vi "Activate Motor.vi"(0 "reference in":refnum<class "PM_Group.lvclass">, 5 "Active Motor":T1, 11 "error in (no error)":errorcluster) -> (4 "reference out":refnum<class "PM_Group.lvclass">, 15 "error out":errorcluster)   [LabVIEW 2019, in "PM_Group.lvclass"]
uses:
  PM_Group.lvclass
  D:/GIT H4000/H4000/src/Device_class/Device.lvclass
  TypeDef/Active Motor.ctl
  TypeDef/Motor N.ctl
  PM_Group.lvclass/PM_Group.ctl
  FPGA/TypeDef/DO index.ctl
  Device_class/Device.lvclass/Device.ctl
  FPGA_API_class/FPGA API.lvclass
  Engine_1DO_2DI_class/Engine_1DO_2DI.lvclass
  Device_class/Device.lvclass
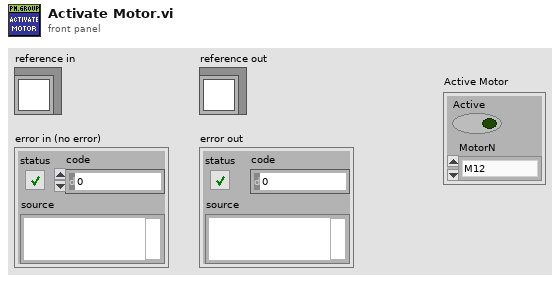
[diagram p1: front panel]
types:
  T1 = typedef "Active Motor.ctl" = cluster{"Active":bool, "MotorN":T2}
  T2 = typedef "Motor N.ctl" = enum16{"M12", "M21", "M24"}
  T3 = typedef "DO index.ctl" = u8
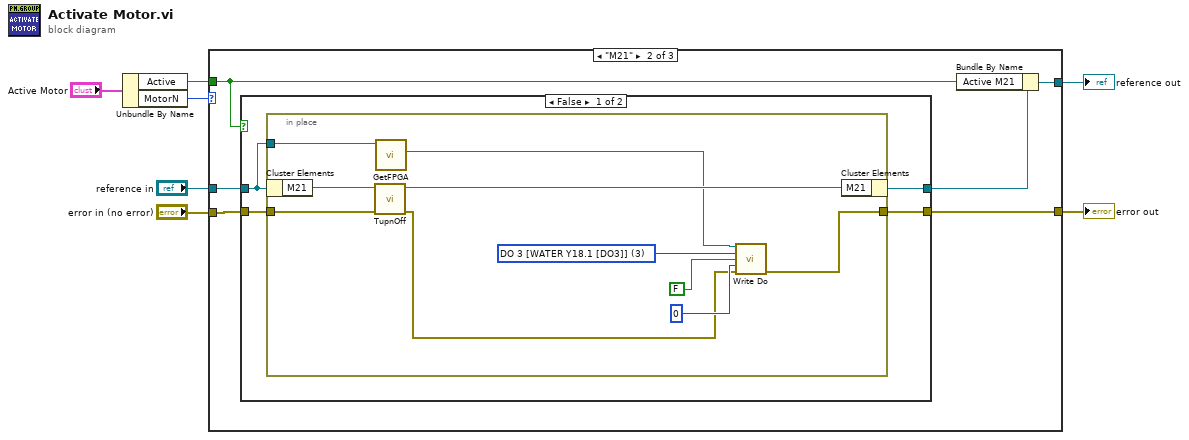
[diagram p0: block diagram]
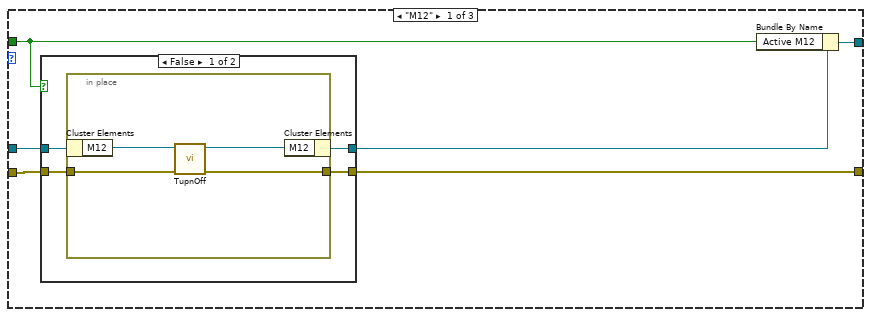
[diagram p2: hidden frame]
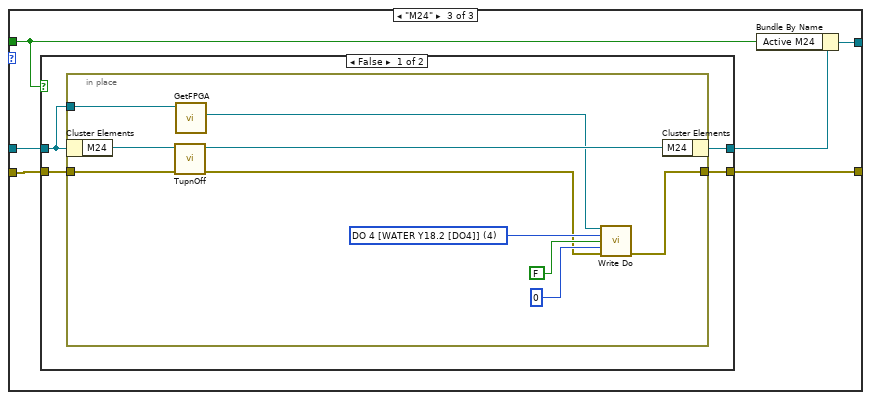
[diagram p5: hidden frame]
diagram:
  n1 = Unbundle By Name("Active Motor") -> ("Active"=w2:bool, "MotorN"=w1:T2)
  n2 = case shown="\"M21\"" w1 {
    tunnel: [w13 w29 w51] -> w7
    tunnel: "error in (no error)" -> [w12 w28 w50]
    tunnel: "reference in" -> [w10 w26 w48]
    tunnel: [w9 w25 w47] -> w4
    tunnel: w2 -> [w8 w24 w46]
    frame "M12" {
      n3 = case shown="False" w8 {
        tunnel: [w17 w22] -> w13
        tunnel: w12 -> [w16 w22]
        tunnel: [w15 w23] -> w11
        tunnel: w10 -> [w14 w23]
        frame False {
          n4 = in-place {
            in-place-border: w16 -> [w19]
            in-place-border: [w18] -> w17
            n5 = in-place-cluster #1(w14) -> ("M12"=w21:refnum<class "Engine_1DO_2DI.lvclass">)
            n6 = call "TupnOff.vi"("error in (no error)"=w19, "Pump_1AI_1DO_2DI in"=w21) -> ("error out"=w18:errorcluster, "Pump_1AI_1DO_2DI out"=w20:refnum<class "Engine_1DO_2DI.lvclass">)  [unwired: 8 in]
            n7 = in-place-cluster #1("M12"=w20) -> (w15:refnum<class "PM_Group.lvclass">)
          }
        }
        frame True {
        }
      }
      n8 = Bundle By Name(cluster=w11, "Active M12"=w8) -> (w9:refnum<class "PM_Group.lvclass">)
    }
    frame "M21" {
      n9 = case shown="False" w24 {
        tunnel: [w33 w44] -> w29
        tunnel: w28 -> [w32 w44]
        tunnel: [w31 w45] -> w27
        tunnel: w26 -> [w30 w45]
        frame False {
          n10 = in-place {
            in-place-border: w32 -> [w41]
            in-place-border: [w36] -> w33
            in-place-border: w30 -> [w35]
            w40 = T3 3 items=["DO 0 [KP1 [DO 0]]", "DO 1 [ON KP2 [DO 1]]", "DO 2 [ON KP3 [DO 2]]", "DO 3 [WATER Y18.1 [DO3]]", "DO 4 [WATER Y18.2 [DO4]]", "DO 5 [KP6 Y29.1 33.7]", "DO 6 [KP7 Y29.2 33.8]", "DO 7 [KP8 Y29.3 33.9]", "DO 8 [KP9 Y29.4  33.12]", "DO 9 [KP10 Y29.5 33.1]", "DO 10 [KP11 Y29.6 33.2]", "DO 11 [KP12 Y29.7  33.13]", "DO 12 [KP13 Y29.8  33.11]", "DO 13 [KP14 Y29.9 33.10]", "DO 14 [KP15 Y29.10  33.6]", "DO 15 [KP16 Y29.11  33.5]", "DO 16 [KP17 Y29.12  33.4]", "DO 17 [KP18 Y29.13 33.3]", "DO 18 [AIR KP19]", "DO 19 [STEP DRIVE EN KP20]", "DO 20 [KP21 Y44.1 OPEN]", "DO 21 [ KP22 Y44.1 CLOSE]", "DO 22 [ KP23 Y44.2 OPEN]", "DO 23", "DO 24 [STEP DRIVE 1]", "DO 25 [STEP DRIVE 2]"] ("#DO")
            n11 = in-place-cluster #2(w30) -> ("M21"=w43:refnum<class "Engine_1DO_2DI.lvclass">)
            n12 = call "TupnOff.vi"("error in (no error)"=w41, "Pump_1AI_1DO_2DI in"=w43) -> ("error out"=w37:errorcluster, "Pump_1AI_1DO_2DI out"=w42:refnum<class "Engine_1DO_2DI.lvclass">)  [unwired: 8 in]
            n13 = call "GetFPGA.vi"("Device in"=w35) -> ("FPGA API.lvclass"=w34:refnum<class "FPGA API.lvclass">)  [unwired: 10 in]
            n14 = call-dynamic "Write Do.vi"("FPGA API in"=w34, "#DO"=w40, "value"=FALSE, "Time uSec"=u32 0, "error in (no error)"=w37) -> ("error out"=w36:errorcluster)  [unwired: 9 in, 1 out]
            n15 = in-place-cluster #2("M21"=w42) -> (w31:refnum<class "PM_Group.lvclass">)
          }
        }
        frame True {
        }
      }
      n16 = Bundle By Name(cluster=w27, "Active M21"=w24) -> (w25:refnum<class "PM_Group.lvclass">)
    }
    frame "M24" {
      n17 = case shown="False" w46 {
        tunnel: [w55 w66] -> w51
        tunnel: w50 -> [w54 w66]
        tunnel: [w53 w67] -> w49
        tunnel: w48 -> [w52 w67]
        frame False {
          n18 = in-place {
            in-place-border: w54 -> [w63]
            in-place-border: [w58] -> w55
            in-place-border: w52 -> [w56]
            w62 = T3 4 items=["DO 0 [KP1 [DO 0]]", "DO 1 [ON KP2 [DO 1]]", "DO 2 [ON KP3 [DO 2]]", "DO 3 [WATER Y18.1 [DO3]]", "DO 4 [WATER Y18.2 [DO4]]", "DO 5 [KP6 Y29.1 33.7]", "DO 6 [KP7 Y29.2 33.8]", "DO 7 [KP8 Y29.3 33.9]", "DO 8 [KP9 Y29.4  33.12]", "DO 9 [KP10 Y29.5 33.1]", "DO 10 [KP11 Y29.6 33.2]", "DO 11 [KP12 Y29.7  33.13]", "DO 12 [KP13 Y29.8  33.11]", "DO 13 [KP14 Y29.9 33.10]", "DO 14 [KP15 Y29.10  33.6]", "DO 15 [KP16 Y29.11  33.5]", "DO 16 [KP17 Y29.12  33.4]", "DO 17 [KP18 Y29.13 33.3]", "DO 18 [AIR KP19]", "DO 19 [STEP DRIVE EN KP20]", "DO 20 [KP21 Y44.1 OPEN]", "DO 21 [ KP22 Y44.1 CLOSE]", "DO 22 [ KP23 Y44.2 OPEN]", "DO 23", "DO 24 [STEP DRIVE 1]", "DO 25 [STEP DRIVE 2]"] ("#DO")
            n19 = in-place-cluster #3(w52) -> ("M24"=w65:refnum<class "Engine_1DO_2DI.lvclass">)
            n20 = call "TupnOff.vi"("error in (no error)"=w63, "Pump_1AI_1DO_2DI in"=w65) -> ("error out"=w59:errorcluster, "Pump_1AI_1DO_2DI out"=w64:refnum<class "Engine_1DO_2DI.lvclass">)  [unwired: 8 in]
            n21 = call "GetFPGA.vi"("Device in"=w56) -> ("FPGA API.lvclass"=w57:refnum<class "FPGA API.lvclass">)  [unwired: 10 in]
            n22 = call-dynamic "Write Do.vi"("FPGA API in"=w57, "#DO"=w62, "value"=FALSE, "Time uSec"=u32 0, "error in (no error)"=w59) -> ("error out"=w58:errorcluster)  [unwired: 9 in, 1 out]
            n23 = in-place-cluster #3("M24"=w64) -> (w53:refnum<class "PM_Group.lvclass">)
          }
        }
        frame True {
        }
      }
      n24 = Bundle By Name(cluster=w49, "Active M24"=w46) -> (w47:refnum<class "PM_Group.lvclass">)
    }
  }
  "error out" <- w7
  "reference out" <- w4
